vi "BASE.LoadConfig.vi"(8 "error in (no error)":errorcluster, 10 "config file path":path, 11 "BASE.Device in":refnum<class "BASE.Device.lvclass">) -> (0 "error out":errorcluster, 3 "BASE.Device out":refnum<class "BASE.Device.lvclass">)   [LabVIEW 2019, in "BASE.Device.lvlib" / "BASE.Device.lvclass"]
uses:
  BASE.Device.lvclass
  BASE.Device.lvclass/BASE.Device.ctl
  BASE/BASE/BASE.lvclass
  <vilib>/Utility/config.llb/NI_LVConfig.lvlib
panel:
  out "class name":string
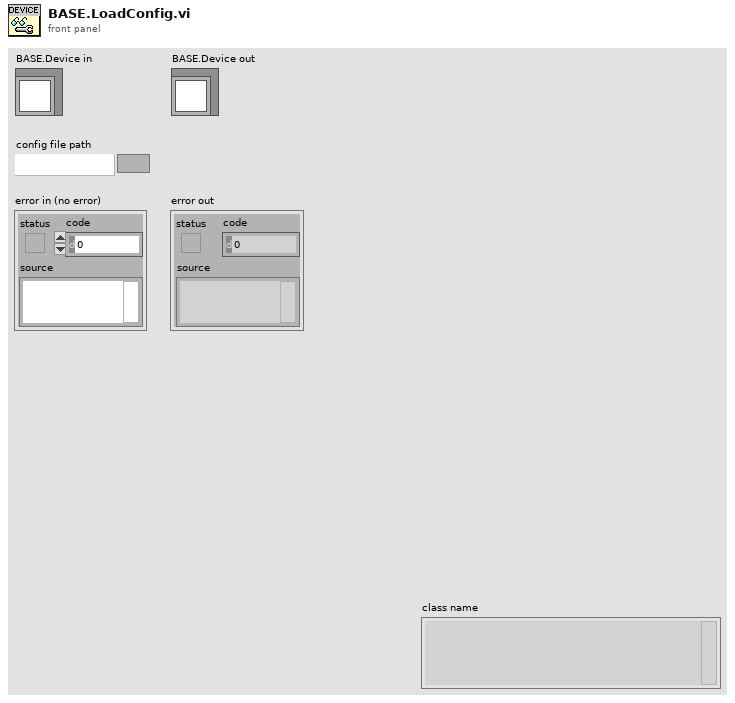
[diagram p1: front panel]
types:
  T1 = typedef "BASE.Device.lvlib/BASE.Device.lvclass/config--cluster.ctl" = cluster{"Connect Timeout":i32, "Check Timeout":i32, "Read Timeout":i32}
  T2 = typedef "NI_LVConfig.lvlib/Config Data RefNum.ctl" = refnum<k1>
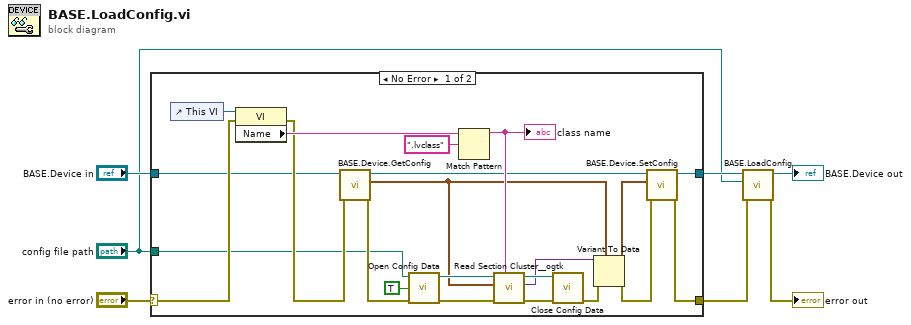
[diagram p0: block diagram]
diagram:
  n1 = case shown="No Error" "error in (no error)" {
    selector: "error in (no error)" -> [w17 w30]
    tunnel: [w9 w30] -> w3
    tunnel: [w12 w29] -> w6
    tunnel: "BASE.Device in" -> [w13 w29]
    tunnel: "config file path" -> [w8 _]
    frame No Error {
      n2 = control-ref of="This VI"() -> (w23:refnum<vi>)
      n3 = property class="VI"(reference=w23, error in=w17) -> (error out=w19:errorcluster, "Name"=w22:string)  [unwired: 1 out]
      n4 = call "BASE.Device.GetConfig.vi"("error in (no error)"=w19, "BASE.Device in"=w13) -> ("error out"=w24:errorcluster, "config"=w15:T1, "BASE.Device out"=w12:refnum<class "BASE.Device.lvclass">)  [unwired: 7 in]
      n5 = call <vilib>:"Open Config Data.vi"("error in (no error)"=w24, "create file if necessary (T)"=TRUE, "configuration file path"=w8) -> ("error out"=w27:errorcluster, "refnum"=w28:T2)  [unwired: 6 in, 1 out]
      n6 = Match Pattern(string=w22, regular expression=".lvclass") -> (before substring=w20:string)  [unwired: 1 in, 3 out]
      "class name" <- w20
      n7 = call <userlib>:"Read Section Cluster__ogtk.vi"("section (optional)"=w20, "error in (no error)"=w27, "Section Formatted Cluster Type"=w15, "refnum"=w28) -> ("error out"=w26:errorcluster, "Section Formatted Cluster"=w16:variant, "dup refnum"=w25:T2)  [unwired: 3 in, 2 out]
      n8 = call <vilib>:"Close Config Data.vi"("error in (no error)"=w26, "refnum"=w25) -> ("error out"=w11:errorcluster)  [unwired: 8 in, 1 out]
      n9 = Variant To Data(error in=w11, type=w15, Variant=w16) -> (data=w14:T1, error out=w10:errorcluster)
      n10 = call "BASE.Device.SetConfig.vi"("error in (no error)"=w10, "config"=w14, "BASE.Device in"=w12) -> ("error out"=w9:errorcluster)  [unwired: 7 in, 1 out]
    }
    frame Error {
    }
  }
  n11 = call-parent "BASE.LoadConfig.vi"("error in (no error)"=w3, "config file path"="config file path", "BASE in"=w6) -> ("error out"=→"error out":errorcluster, "BASE out"=→"BASE.Device out":refnum<class "BASE.Device.lvclass">)  [unwired: 7 in]
